vi "Modules - Data Logging.vi"(8 "error in":errorcluster) -> (0 "error out":errorcluster)   [LabVIEW 2019]
uses:
  Controls/Error Log-State.ctl
  Controls/eFGV States.ctl
types:
  T1 = typedef "Error Log-State.ctl" = enum16{"Init", "Idle", "Write", "Exit"}
  T2 = enum16{"open", "replace", "create", "open or create", "replace or create", "replace or create with confirmation"}
  T3 = typedef "eFGV States.ctl" = enum16{"Init", "Read", "Write", "Exit"}
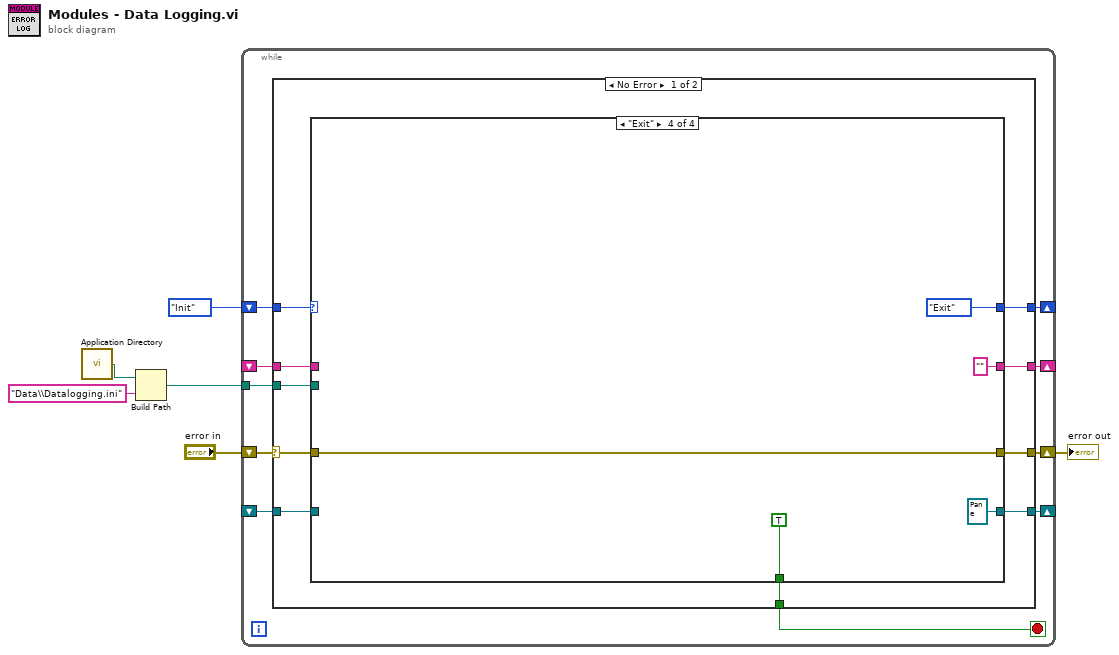
[diagram p0: block diagram]
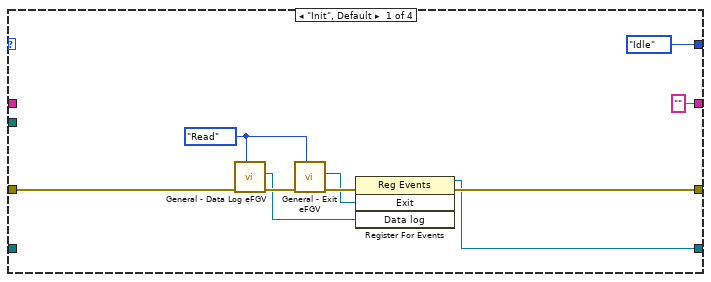
[diagram p2: hidden frame]
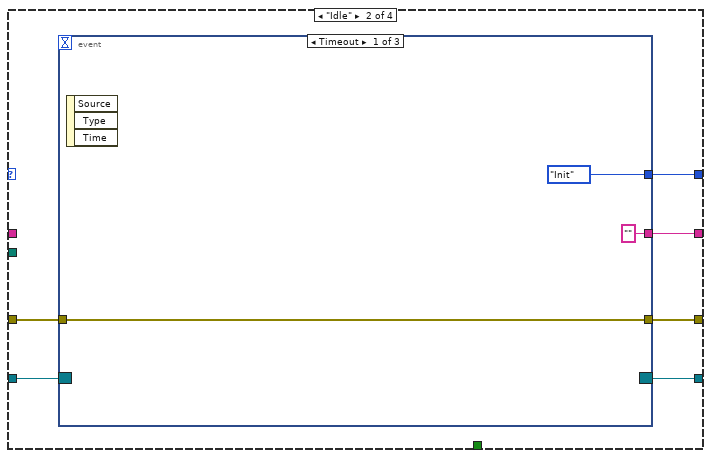
[diagram p3: hidden frame]
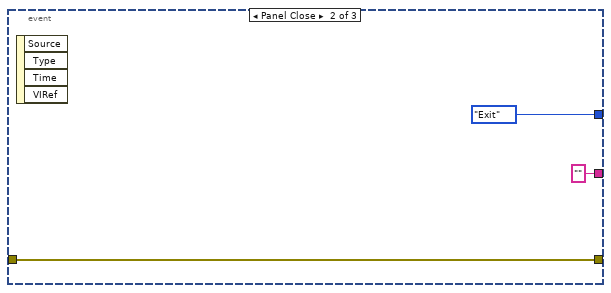
[diagram p4: hidden frame]
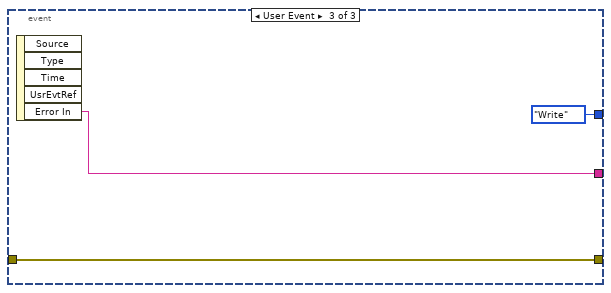
[diagram p5: hidden frame]
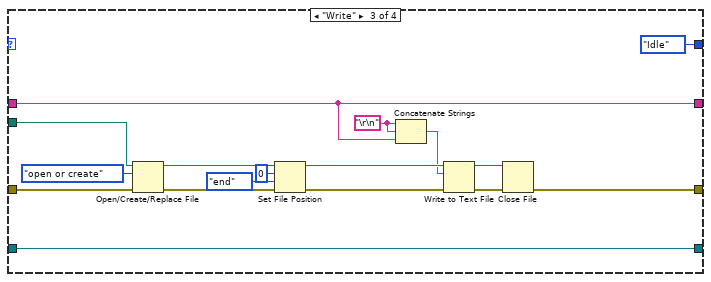
[diagram p6: hidden frame]
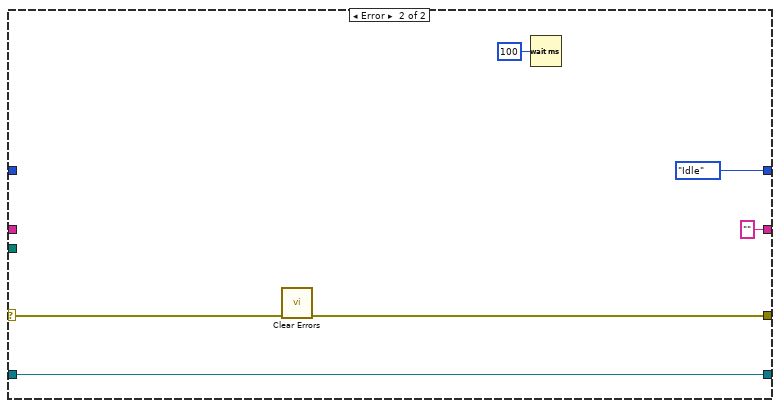
[diagram p7: hidden frame]
diagram:
  n1 = call <vilib>:"Application Directory.vi"() -> ("Application Directory"=w3:path)
  n2 = Build Path(base path=w3, name or relative path="Data\\Datalogging.ini") -> (appended path=w1:path)
  n3 = while {
    shift-right: [w15] -> w5
    shift-left: "error in" -> [w16]
    shift-right: [w13] -> _
    shift-left: Error_Log-State."Init" ("Enum") -> [w14]
    shift-right: [w11] -> _
    shift-left: _ -> [w10]
    shift-right: [w9] -> _
    shift-left: _ -> [w8]
    tunnel: w1 -> [w7]
    stop <- w12 stop-if-true
    n4 = case shown="No Error" w16 {
      selector: w16 -> [w25 w79]
      tunnel: [w24 w78] -> w15
      tunnel: w14 -> [w26 _]
      tunnel: [w23 Error_Log-State."Idle" ("Enum")] -> w13
      tunnel: [w22 _] -> w12
      tunnel: [w21 w76] -> w11
      tunnel: w10 -> [w20 w76]
      tunnel: [w19 "" ("Error In")] -> w9
      tunnel: w8 -> [w18 _]
      tunnel: w7 -> [w17 _]
      frame No Error {
        n5 = case shown="\"Exit\"" w26 {
          tunnel: w25 -> [w30 w40 w65 w72]
          tunnel: [w34 w42 w62 w72] -> w24
          tunnel: [Error_Log-State."Idle" ("Enum") w41 Error_Log-State."Idle" ("Enum") Error_Log-State."Exit" ("Enum")] -> w23
          tunnel: [_ _ _ TRUE] -> w22
          tunnel: [w33 w38 w68 refnum<event-registration> refnum ("Event Registration Refnum")] -> w21
          tunnel: w20 -> [_ w39 w68 _]
          tunnel: ["" ("Error In") w37 w54 "" ("Error In")] -> w19
          tunnel: w18 -> [_ _ w54 _]
          tunnel: w17 -> [_ _ w64 _]
          frame "Init", Default {
            w28 = eFGV_States."Read" ("eFGV States")
            n6 = call "General - Data Log eFGV.vi"("eFGV States"=w28, "error in (no error)"=w30) -> ("error out"=w29:errorcluster, "Data log"=w27:refnum<user-event>)  [unwired: 7 in, 1 out]
            n7 = call "General - Exit eFGV.vi"("eFGV States"=w28, "error in (no error)"=w29) -> ("error out"=w36:errorcluster, "Exit"=w35:refnum<user-event>)  [unwired: 7 in, 1 out]
            n8 = register-events(error in=w36, w35, w27) -> (reference out=w33:refnum<event-registration>, error out=w34:errorcluster)  [unwired: 1 in]
          }
          frame "Idle" {
            n9 = event shown="[0] Timeout" {
              selector: w39 -> [_ _ _]
              dyn-events: [_ _ _] -> w38
              timeout: _ -> [_ _ _]
              tunnel: w40 -> [w45 w48 w51]
              tunnel: [w45 w48 w51] -> w42
              tunnel: [Error_Log-State."Init" ("Enum") Error_Log-State."Exit" ("Enum") Error_Log-State."Write" ("Enum")] -> w41
              tunnel: ["" ("Error In") "" ("Error In") w50] -> w37
              event Timeout {
                n10 = event-data() -> ()  [unwired: 1 in, 3 out]
              }
              event Panel Close {
                n11 = event-data() -> ()  [unwired: 1 in, 4 out]
              }
              event User Event {
                n12 = event-data() -> ("Error In"=w50:string)  [unwired: 1 in, 4 out]
              }
            }
          }
          frame "Write" {
            w52 = "\r\n"
            n13 = Open/Create/Replace File(file path (use dialog)=w64, error in=w65, operation (0:open)=T2."open or create") -> (refnum out=w56:refnum<file>, error out=w58:errorcluster)  [unwired: 3 in, 1 out]
            n14 = Set File Position(offset (in bytes) (0)=i64 0, refnum=w56, from (0:start)=enum16{"start", "end", "current"}."end", error in=w58) -> (refnum out=w55:refnum<file>, error out=w57:errorcluster)
            n15 = Concatenate Strings(w52, w52, w54) -> (w53:string)
            n16 = Write to Text File(file (use dialog)=w55, text=w53, error in=w57) -> (refnum out=w61:refnum<file>, error out=w66:errorcluster)  [unwired: 1 in, 1 out]
            n17 = Close File(refnum=w61, error in=w66) -> (error out=w62:errorcluster)  [unwired: 1 out]
          }
          frame "Exit" {
          }
        }
      }
      frame Error {
        n18 = call <vilib>:"Clear Errors.vi"("error in (no error)"=w79) -> ("error out"=w78:errorcluster)  [unwired: 5 in, 1 out]
        n19 = Wait (ms)(milliseconds to wait=u32 100) -> ()  [unwired: 1 out]
      }
    }
  }
  "error out" <- w5
